vi "Dictionary to X and Y Arrays.vi"(8 "error in (no error)":errorcluster, 11 "Results (Dictionary)":cluster{"key":string, "value":dbl}[](array[cluster])) -> (0 "error out":errorcluster, 2 "Data":dbl[](array[numeric]), 3 "Data 2":dbl[](array[numeric]))   [LabVIEW 2016, in "Transport.lvclass"]
uses:
  Transport.lvclass
  <userlib>/LevyLab/Lockin-Multichannel/Instrument.Lockin/Typedefs/Results Type--Enum.ctl
  <userlib>/LevyLab/Lockin-Multichannel/Instrument.Lockin/Instrument.Lockin.lvclass
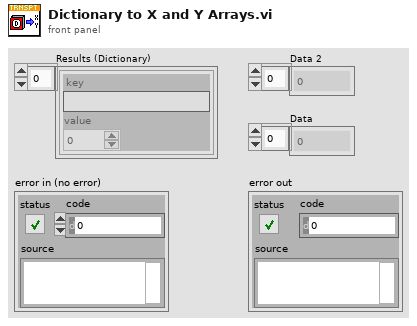
[diagram p1: front panel]
types:
  T1 = typedef "Instrument.Lockin.lvclass/Results Type--Enum.ctl" = enum16{"X", "Y", "R", "Theta", "Mean"}
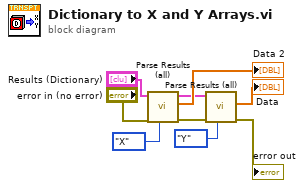
[diagram p0: block diagram]
diagram:
  n1 = call <userlib>:"Parse Results (all).vi"("Type"=Results_Type--Enum."X", "error in (no error)"="error in (no error)", "Results (Dictionary)"="Results (Dictionary)") -> ("error out"=w6:errorcluster, "Data"=→"Data 2":dbl[], "Results (Dictionary)"=w3:cluster{"key":string, "value":dbl}[])  [unwired: 5 in, 1 out]
  n2 = call <userlib>:"Parse Results (all).vi"("Type"=Results_Type--Enum."Y", "error in (no error)"=w6, "Results (Dictionary)"=w3) -> ("error out"=→"error out":errorcluster, "Data"=→"Data":dbl[])  [unwired: 5 in, 2 out]
